vi "folderizer.vi"() -> ()   [LabVIEW 2012]
panel:
  out "error out":errorcluster
  out "Copying progress (%)":dbl(slide) scale=0.0..100.0
  in  "Destination folder":path
  in  "Source folder":path
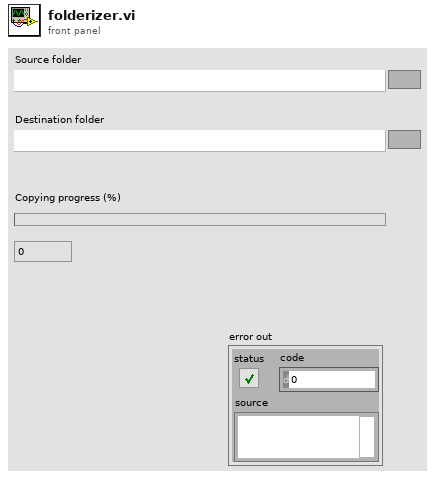
[diagram p1: front panel]
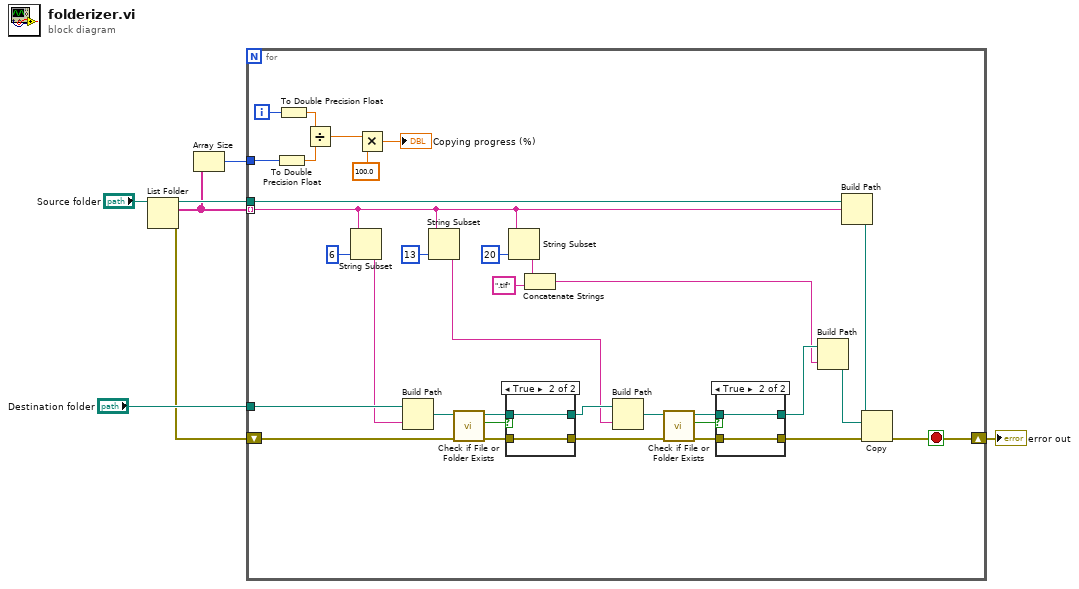
[diagram p0: block diagram]
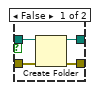
[diagram p2: hidden frame]
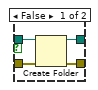
[diagram p3: hidden frame]
diagram:
  n1 = List Folder(path="Source folder") -> (path out=w6:path, filenames=w3:string[], error out=w4:errorcluster)  [unwired: 3 in, 1 out]
  n2 = Array Size(array=w3) -> (size(s)=w2:i32)
  n3 = for {
    tunnel: w3 -> [w18] mode=indexing
    tunnel: w6 -> [w19]
    tunnel: "Destination folder" -> [w40]
    shift-right: [w15] -> w1
    shift-left: w4 -> [w38]
    tunnel: w2 -> [w13]
    i -> [w14]
    stop <- w15 stop-if-true
    n4 = To Double Precision Float(number=w13) -> (double precision float=w12:dbl)
    n5 = To Double Precision Float(number=w14) -> (double precision float=w11:dbl)
    n6 = Divide(x=w11, y=w12) -> (x/y=w10:dbl)
    n7 = String Subset(string=w18, length (rest)=6 ("length (rest)")) -> (substring=w28:string)  [unwired: 1 in]
    n8 = Multiply(x=w10, y=100.0) -> (x*y=→"Copying progress (%)":dbl)
    n9 = Build Path(base path=w40, name or relative path=w28) -> (appended path=w39:path)
    n10 = String Subset(string=w18, length (rest)=13 ("length (rest)")) -> (substring=w25:string)  [unwired: 1 in]
    n11 = call <vilib>:"Check if File or Folder Exists.vi"("error in (no error)"=w38, "path"=w39) -> ("error out"=w36:errorcluster, "file or folder exists?"=w37:bool, "dup path"=w35:path)  [unwired: 7 in]
    n12 = case shown="True" w37 {
      tunnel: w36 -> [w51 w52]
      tunnel: w35 -> [w50 w53]
      tunnel: [w49 w52] -> w30
      tunnel: [w48 w53] -> w29
      frame False {
        n13 = Create Folder(path (use dialog)=w50, error in=w51) -> (created path=w48:path, error out=w49:errorcluster)  [unwired: 1 in, 1 out]
      }
      frame True {
      }
    }
    n14 = String Subset(string=w18, length (rest)=20 ("length (rest)")) -> (substring=w23:string)  [unwired: 1 in]
    n15 = Concatenate Strings(w23, ".tif" ("string")) -> (w21:string)
    n16 = Build Path(base path=w29, name or relative path=w25) -> (appended path=w34:path)
    n17 = call <vilib>:"Check if File or Folder Exists.vi"("error in (no error)"=w30, "path"=w34) -> ("error out"=w32:errorcluster, "file or folder exists?"=w33:bool, "dup path"=w31:path)  [unwired: 7 in]
    n18 = case shown="True" w33 {
      tunnel: w32 -> [w45 w46]
      tunnel: w31 -> [w44 w47]
      tunnel: [w43 w46] -> w20
      tunnel: [w42 w47] -> w22
      frame False {
        n19 = Create Folder(path (use dialog)=w44, error in=w45) -> (created path=w42:path, error out=w43:errorcluster)  [unwired: 1 in, 1 out]
      }
      frame True {
      }
    }
    n20 = Build Path(base path=w22, name or relative path=w21) -> (appended path=w16:path)
    n21 = Build Path(base path=w19, name or relative path=w18) -> (appended path=w17:path)
    n22 = Copy(8:w20, 10:w16, 11:w17) -> (0:w15:errorcluster)  [unwired: 2 in, 2 out]
  }
  "error out" <- w1
